vi "setUp.vi"(8 "error in (no error)":errorcluster, 11 "reference in":refnum<class "Multi Consumer Test Case.lvclass">) -> (0 "error out":errorcluster, 3 "reference out":refnum<class "Multi Consumer Test Case.lvclass">)   [LabVIEW 2027, in "Multi Consumer Test Case.lvclass"]
doc: "setUp runs prior to the test method during test execution. Use this method to initialize any object data required by your tests."
uses:
  Multi Consumer Test Case.lvclass
  C:/Program Files/National Instruments/LabVIEW 2027/vi.lib/addons/_JKI Toolkits/VI Tester/TestCase.llb/TestCase.lvclass
  Producer/Abstract Producer/Abstract Producer.lvclass
  Parameters/Abstract Init Parameters/Abstract Init Parameters.lvclass
  Message Queue/Message Queue/Message Queue.lvclass
  C:/NetCore/niveristand-custom-device-message-library/Source/Message Queue/Abstract Message Queue/Abstract Message Queue.lvclass
  Support/Consumers/Test Consumer/Test Consumer.lvclass
  C:/NetCore/niveristand-custom-device-message-library/Source/Consumer/Abstract Consumer/Abstract Consumer.lvclass
  Support/Message String Action.ctl
  Support/Message List Action.ctl
  Multi Consumer Test Case.lvclass/Multi Consumer Test Case.ctl
  <vilib>/addons/_JKI Toolkits/VI Tester/TestCase.llb/TestCase.lvclass
  Consumer/Abstract Consumer/Abstract Consumer.lvclass
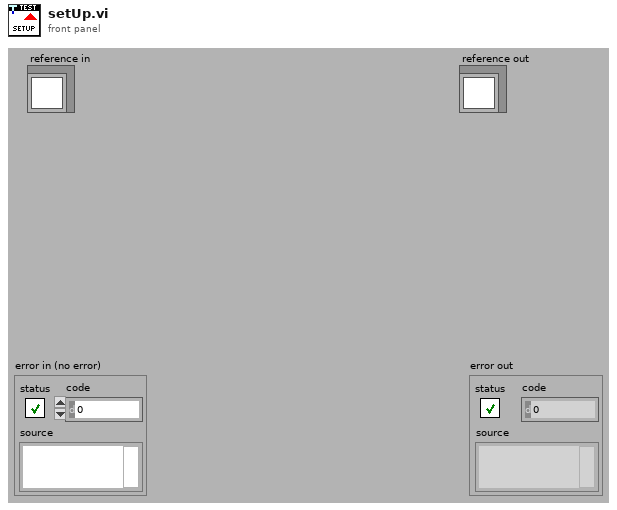
[diagram p1: front panel]
types:
  T1 = typedef "Message List Action.ctl" = enum16{"Get", "Add", "Reset"}
  T2 = typedef "Message String Action.ctl" = enum16{"Get String", "Set String", "Reset"}
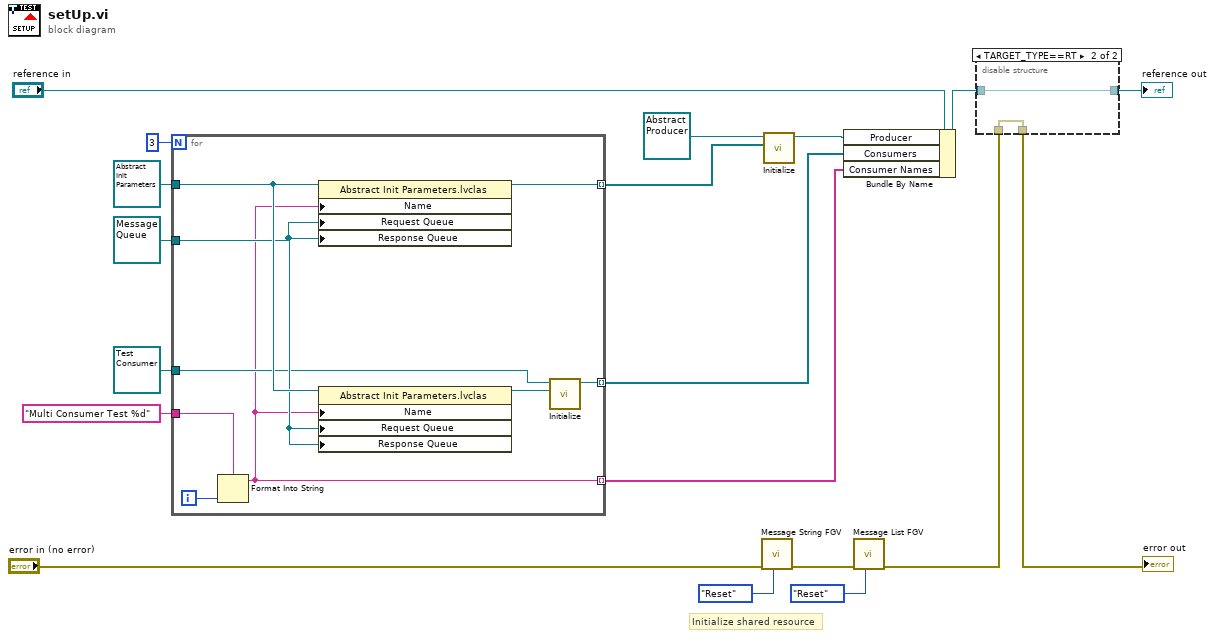
[diagram p0: block diagram]
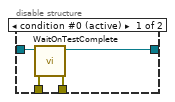
[diagram p2: hidden frame]
diagram:
  # "Initialize shared resource"
  n1 = for {
    N: 3 -> [_]
    tunnel: refnum<class "Message Queue.lvclass"> refnum ("Messaging.lvlib:Message Queue.lvlib:Message Queue.lvclass") -> [w26]
    tunnel: refnum<class "Abstract Init Parameters.lvclass"> refnum ("Message Queue Library.lvlib:Abstract Init Parameters.lvclass") -> [w28]
    tunnel: [w27] -> w13 mode=indexing
    tunnel: refnum<class "Test Consumer.lvclass"> refnum ("Reflected Name Consumer.lvclass") -> [w24]
    tunnel: [w23] -> w8 mode=indexing
    tunnel: "Multi Consumer Test %d" ("Name") -> [w22]
    tunnel: [w20] -> w7 mode=indexing
    i -> [w21]
    n2 = Format Into String(format string=w22, w21) -> (resulting string=w20:string)  [unwired: 2 in, 1 out]
    n3 = property class="Abstract Init Parameters.lvclas"(reference=w28, "Name"=w20, "Request Queue"=w26, "Response Queue"=w26) -> (reference out=w27:refnum<class "Abstract Init Parameters.lvclass">)  [unwired: 1 in, 1 out]
    n4 = property class="Abstract Init Parameters.lvclas"(reference=w28, "Name"=w20, "Request Queue"=w26, "Response Queue"=w26) -> (reference out=w25:refnum<class "Abstract Init Parameters.lvclass">)  [unwired: 1 in, 1 out]
    n5 = call "Initialize.vi"("Parameters in"=w25, "Abstract Consumer in"=w24) -> ("Abstract Consumer out"=w23:refnum<class "Test Consumer.lvclass">)  [unwired: 8 in, 1 out]
  }
  n6 = call "Message String FGV.vi"("Action"=Message_String_Action."Reset", "error in (no error)"="error in (no error)") -> ("error out"=w6:errorcluster)  [unwired: 8 in, 1 out]
  n7 = call "Initialize.vi"("Parameters in"=w13, "Abstract Producer in"=refnum<class "Abstract Producer.lvclass"> refnum ("Messaging.lvlib:Producer.lvlib:Abstract Producer.lvclass")) -> ("Abstract Producer out"=w9:refnum<class "Abstract Producer.lvclass">)  [unwired: 8 in, 1 out]
  n8 = Bundle By Name(cluster="reference in", "Producer"=w9, "Consumers"=w8, "Consumer Names"=w7) -> (w16:refnum<class "Multi Consumer Test Case.lvclass">)
  n9 = call "Message List FGV.vi"("Action (Get)"=Message_List_Action."Reset", "error in (no error)"=w6) -> ("error out"=w4:errorcluster)  [unwired: 8 in, 1 out]
  n10 = disable-structure shown="TARGET_TYPE==RT" {
    disable-tunnel: w4 -> [w32 w33]
    disable-tunnel: [w31 w33] -> w19
    disable-tunnel: [w30 w34] -> w17
    disable-tunnel: w16 -> [w29 w34]
    frame condition #0 (active) {
      n11 = call <vilib>:"WaitOnTestComplete.vi"("error in (no error)"=w32, "TestCase in"=w29) -> ("error out"=w31:errorcluster, "TestCase out"=w30:refnum<class "Multi Consumer Test Case.lvclass">)  [unwired: 8 in]
    }
    frame condition #1 {
    }
  }
  "error out" <- w19
  "reference out" <- w17
